vi "HeatFlow Conf Results.vi"(8 "error in":errorcluster, 9 "All signals?":bool, 11 "HW Cfg In":T2) -> (0 "error out":errorcluster, 2 "HeatFlowRes Cfg":T1, 3 "HW Cfg Out":T2)   [LabVIEW 2019, in "Acquisition.lvlib"]
uses:
  Acquisition.lvlib
  HeatFlow HW Cfg.ctl
  Logging/HeatFlow/HeatFlow Res Cfg.ctl
  Logging/HeatFlow/HeatFlow Results States.ctl
  Logging/Logging.lvlib
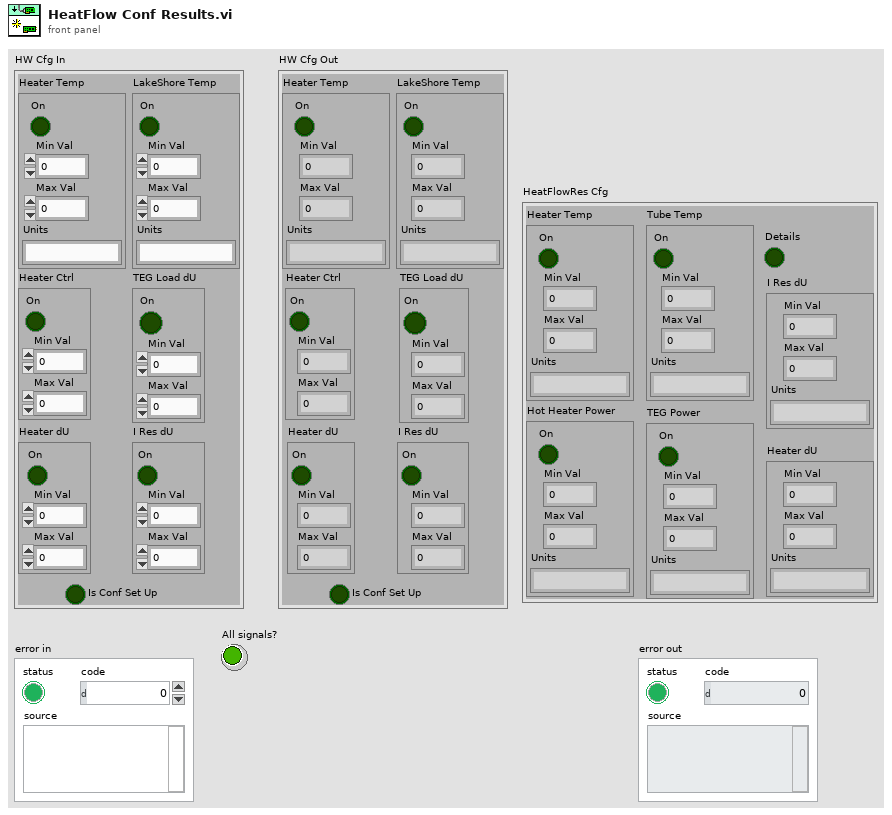
[diagram p1: front panel]
types:
  T1 = typedef "Logging.lvlib/HeatFlow Res Cfg.ctl" = cluster{"Heater Temp":cluster{"On":bool, "Min Val":dbl, "Max Val":dbl, "Units":string}, "Tube Temp":cluster{"On":bool, "Min Val":dbl, "Max Val":dbl, "Units":string}, "Hot Heater Power":cluster{"On":bool, "Min Val":dbl, "Max Val":dbl, "Units":string}, "TEG Power":cluster{"On":bool, "Min Val":dbl, "Max Val":dbl, "Units":string}, "Details":bool, "Heater dU":cluster{"Min Val":dbl, "Max Val":dbl, "Units":string}, "I Res dU":cluster{"Min Val":dbl, "Max Val":dbl, "Units":string}}
  T2 = typedef "Acquisition.lvlib/HeatFlow HW Cfg.ctl" = cluster{"Heater Temp":cluster{"On":bool, "Min Val":dbl, "Max Val":dbl, "Units":string}, "LakeShore Temp":cluster{"On":bool, "Min Val":dbl, "Max Val":dbl, "Units":string}, "Heater Ctrl":cluster{"On":bool, "Min Val":dbl, "Max Val":dbl}, "TEG Load dU":cluster{"On":bool, "Min Val":dbl, "Max Val":dbl}, "Heater dU":cluster{"On":bool, "Min Val":dbl, "Max Val":dbl}, "I Res dU":cluster{"On":bool, "Min Val":dbl, "Max Val":dbl}, "Is Conf Set Up":bool}
  T3 = typedef "Logging.lvlib/HeatFlow Results States.ctl" = enum16{"Start", "Timestamp", "Heater Temp", "Tube Temp", "Heater Power", "TEG Power", "Details", "End"}
  T4 = cluster{"On":bool, "Min Val":dbl, "Max Val":dbl, "Units":string}
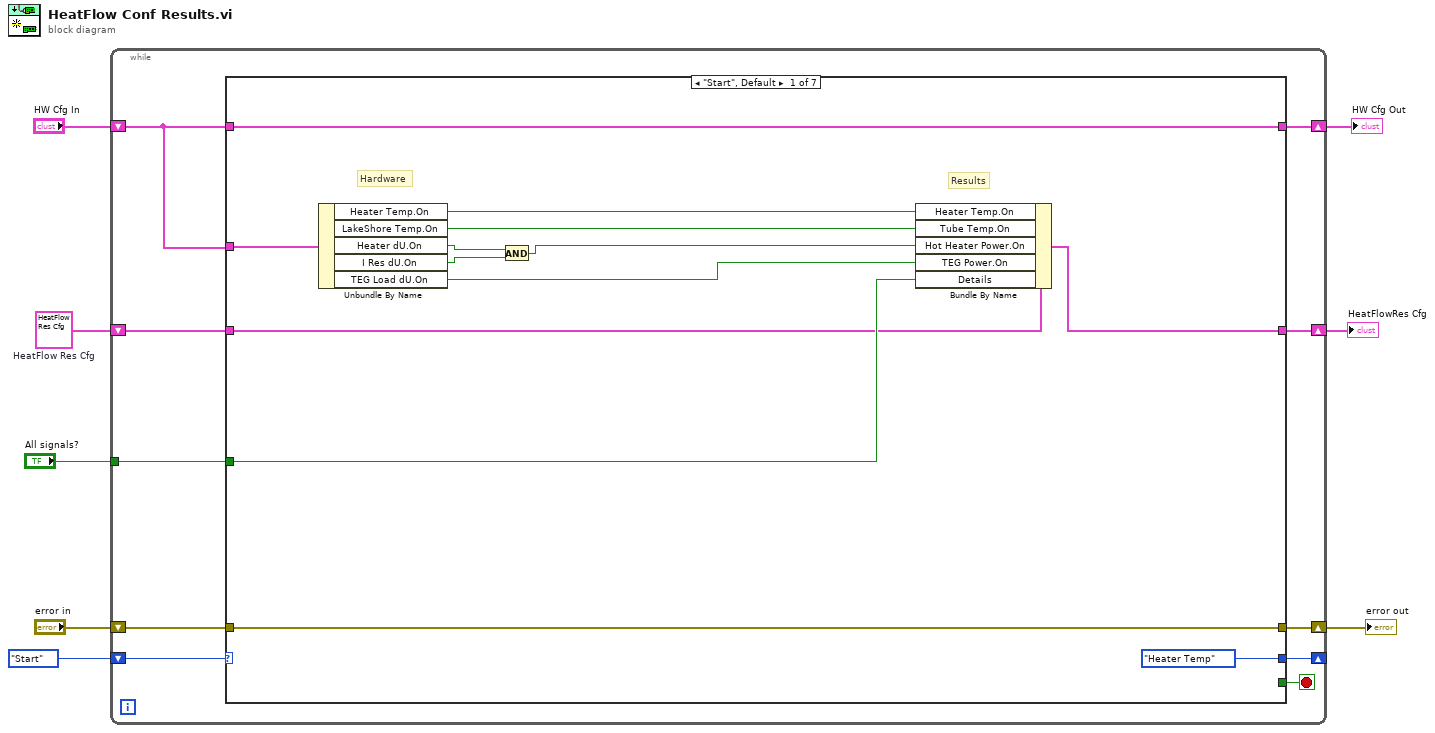
[diagram p0: block diagram]
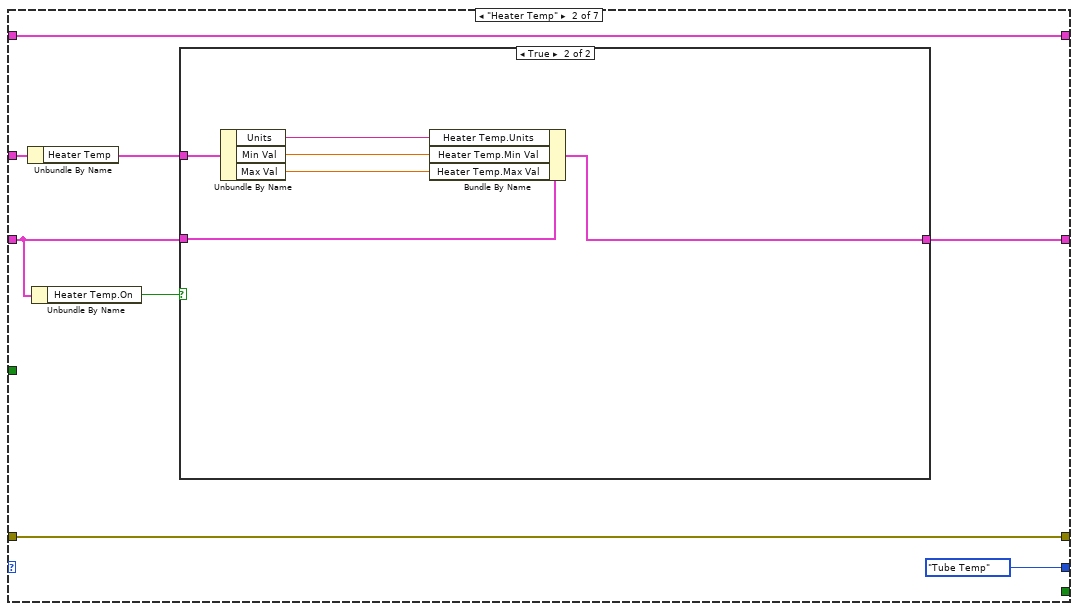
[diagram p2: hidden frame]
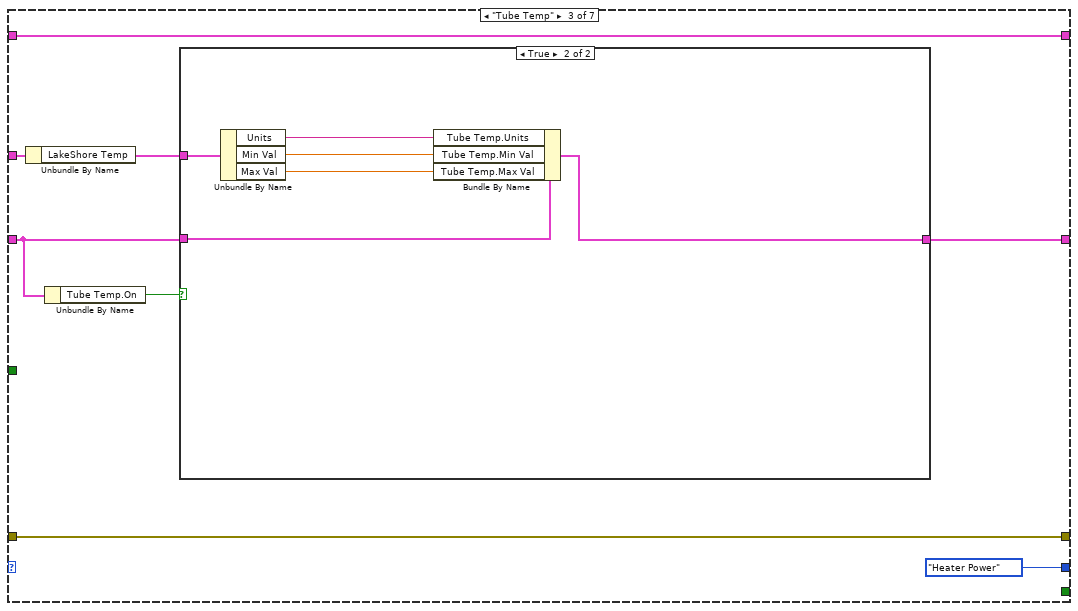
[diagram p4: hidden frame]
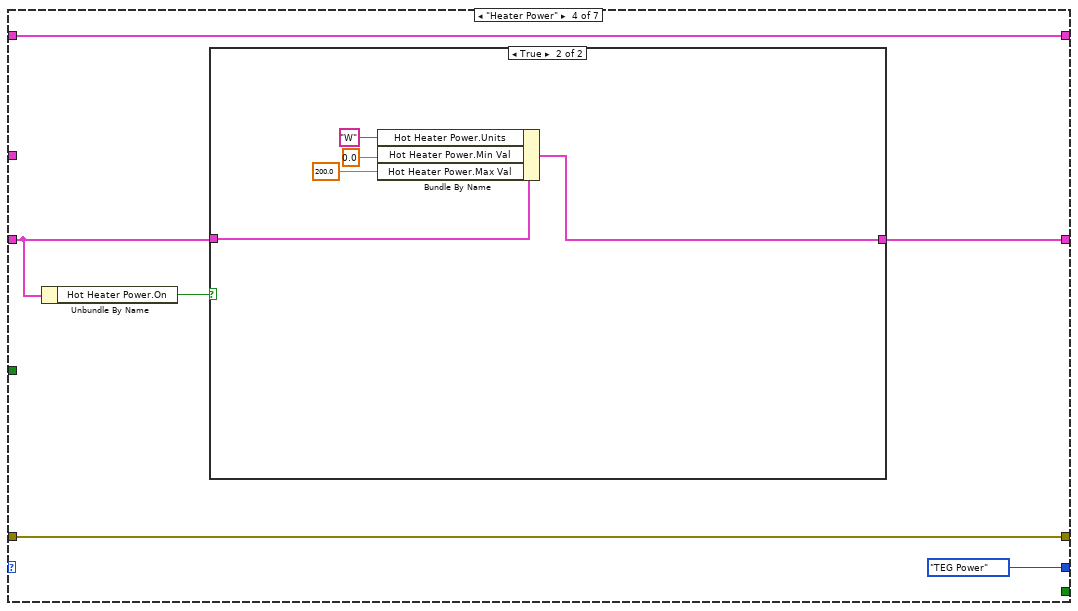
[diagram p6: hidden frame]
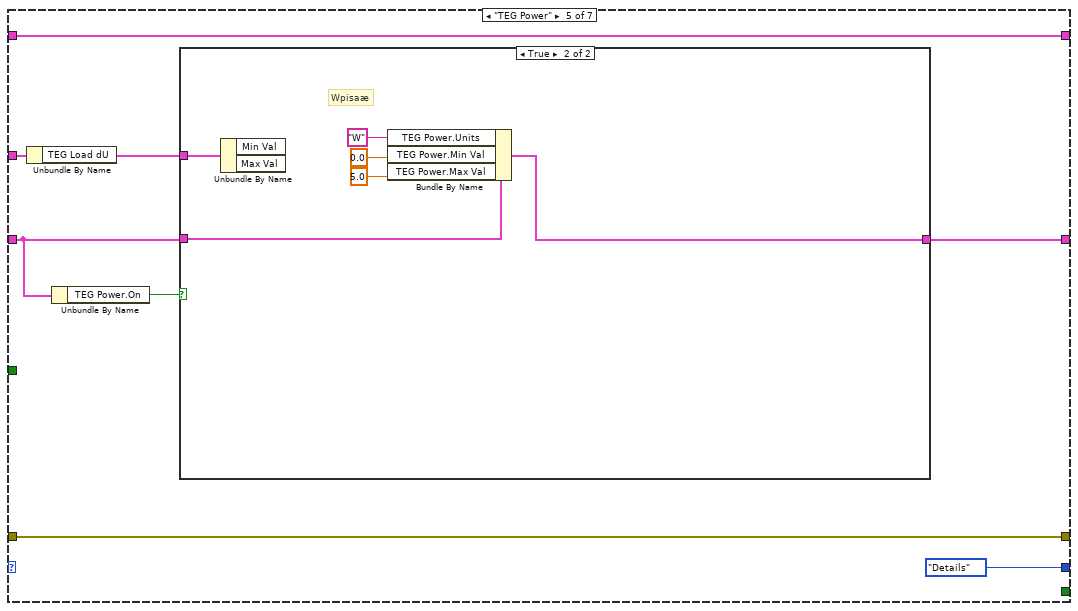
[diagram p8: hidden frame]
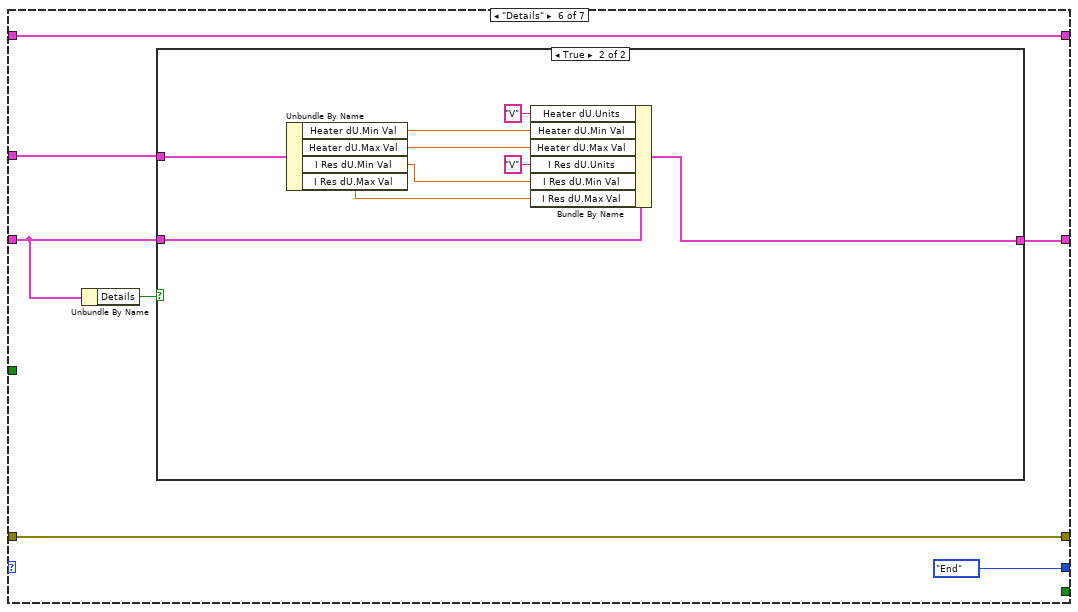
[diagram p10: hidden frame]
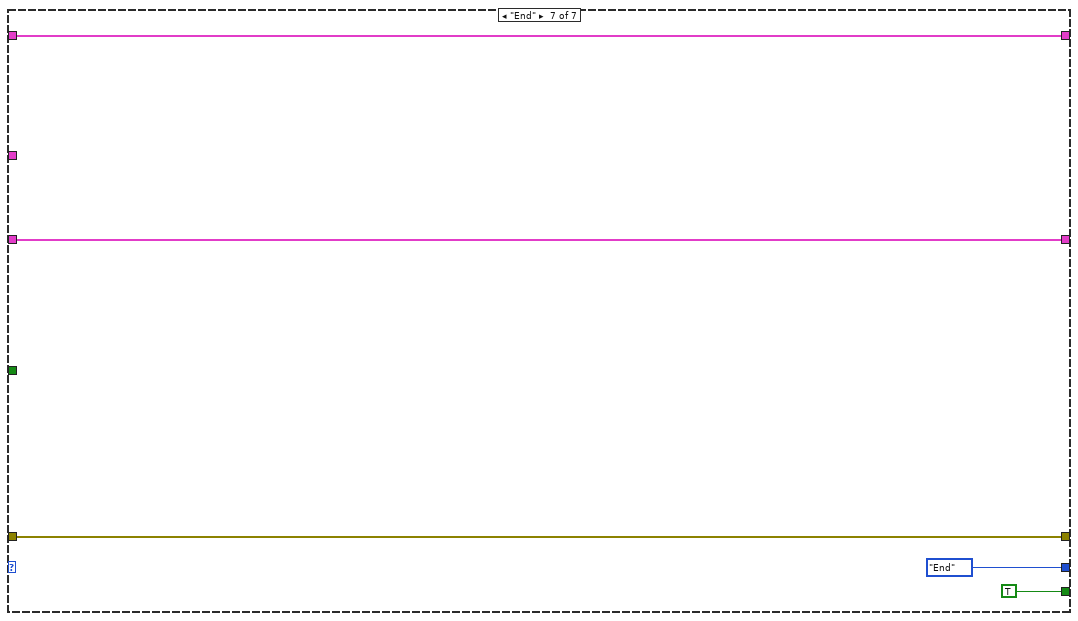
[diagram p12: hidden frame]
diagram:
  w2 = T1 {"Heater Temp"={"On"=FALSE, "Min Val"=0.0, "Max Val"=0.0, "Units"=""}, "Tube Temp"={"On"=FALSE, "Min Val"=0.0, "Max Val"=0.0, "Units"=""}, "Hot Heater Power"={"On"=FALSE, "Min Val"=0.0, "Max Val"=0.0, "Units"=""}, "TEG Power"={"On"=FALSE, "Min Val"=0.0, "Max Val"=0.0, "Units"=""}, "Details"=FALSE, "Heater dU"={"Min Val"=0.0, "Max Val"=0.0, "Units"=""}, "I Res dU"={"Min Val"=0.0, "Max Val"=0.0, "Units"=""}}  # HeatFlow Res Cfg
  n1 = while {
    shift-right: [w17] -> _
    shift-left: HeatFlow_Results_States."Start" ("Results") -> [w18]
    shift-right: [w16] -> w3
    shift-left: "HW Cfg In" -> [w11]
    shift-right: [w14] -> w5
    shift-left: "error in" -> [w15]
    tunnel: "All signals?" -> [w12]
    shift-right: [w9] -> w1
    shift-left: w2 -> [w10]
    stop <- w13 stop-if-true
    n2 = case shown="\"Start\", Default" w18 {
      tunnel: [HeatFlow_Results_States."Heater Temp" ("Results") HeatFlow_Results_States."Tube Temp" ("Results") HeatFlow_Results_States."Heater Power" ("Results") HeatFlow_Results_States."TEG Power" ("Results") HeatFlow_Results_States."Details" ("Results") HeatFlow_Results_States."End" ("Results") HeatFlow_Results_States."End" ("Results")] -> w17
      tunnel: w11 -> [w21 w33 w48 w63 w75 w93 w110]
      tunnel: [w21 w33 w48 w63 w75 w93 w110] -> w16
      tunnel: w15 -> [w31 w32 w47 w62 w74 w94 w109]
      tunnel: [w31 w32 w47 w62 w74 w94 w109] -> w14
      tunnel: w10 -> [w20 w36 w51 w65 w78 w91 w106]
      tunnel: [_ _ _ _ _ _ TRUE] -> w13
      tunnel: w12 -> [w28 _ _ _ _ _ _]
      tunnel: w11 -> [w27 w39 w54 _ w81 w92 _]
      tunnel: [w19 w34 w49 w64 w76 w89 w106] -> w9
      frame "Start", Default {
        # "Results"
        # "Hardware"
        n3 = Unbundle By Name(w27) -> ("Heater Temp.On"=w30:bool, "LakeShore Temp.On"=w29:bool, "Heater dU.On"=w25:bool, "I Res dU.On"=w24:bool, "TEG Load dU.On"=w22:bool)
        n4 = And(x=w25, y=w24) -> (x .and. y?=w23:bool)
        n5 = Bundle By Name(cluster=w20, "Heater Temp.On"=w30, "Tube Temp.On"=w29, "Hot Heater Power.On"=w23, "TEG Power.On"=w22, "Details"=w28) -> (w19:T1)
      }
      frame "Heater Temp" {
        n6 = Unbundle By Name(w39) -> ("Heater Temp"=w38:T4)
        n7 = Unbundle By Name(w36) -> ("Heater Temp.On"=w37:bool)
        n8 = case shown="True" w37 {
          tunnel: w38 -> [_ w46]
          tunnel: w36 -> [w40 w42]
          tunnel: [w40 w41] -> w34
          frame False {
            # "Inlet temperature measurement is off."
          }
          frame True {
            # "Inlet temperature measurement is on."
            n9 = Unbundle By Name(w46) -> ("Units"=w45:string, "Min Val"=w44:dbl, "Max Val"=w43:dbl)
            n10 = Bundle By Name(cluster=w42, "Heater Temp.Units"=w45, "Heater Temp.Min Val"=w44, "Heater Temp.Max Val"=w43) -> (w41:T1)
          }
        }
      }
      frame "Tube Temp" {
        n11 = Unbundle By Name(w54) -> ("LakeShore Temp"=w53:T4)
        n12 = Unbundle By Name(w51) -> ("Tube Temp.On"=w52:bool)
        n13 = case shown="True" w52 {
          tunnel: w53 -> [_ w61]
          tunnel: w51 -> [w55 w60]
          tunnel: [w55 w56] -> w49
          frame False {
            # "Inlet temperature measurement is off."
          }
          frame True {
            # "Inlet temperature measurement is on."
            n14 = Unbundle By Name(w61) -> ("Units"=w59:string, "Min Val"=w58:dbl, "Max Val"=w57:dbl)
            n15 = Bundle By Name(cluster=w60, "Tube Temp.Units"=w59, "Tube Temp.Min Val"=w58, "Tube Temp.Max Val"=w57) -> (w56:T1)
          }
        }
      }
      frame "Heater Power" {
        n16 = Unbundle By Name(w65) -> ("Hot Heater Power.On"=w67:bool)
        n17 = case shown="True" w67 {
          tunnel: w65 -> [w68 w73]
          tunnel: [w68 w69] -> w64
          frame False {
            # "Inlet temperature measurement is off."
          }
          frame True {
            # "Inlet temperature measurement is on."
            n18 = Bundle By Name(cluster=w73, "Hot Heater Power.Units"="W" ("Units"), "Hot Heater Power.Min Val"=0.0 ("Min Val"), "Hot Heater Power.Max Val"=200.0 ("Max Val")) -> (w69:T1)
          }
        }
      }
      frame "TEG Power" {
        n19 = Unbundle By Name(w81) -> ("TEG Load dU"=w80:cluster{"On":bool, "Min Val":dbl, "Max Val":dbl})
        n20 = Unbundle By Name(w78) -> ("TEG Power.On"=w79:bool)
        n21 = case shown="True" w79 {
          tunnel: w80 -> [_ w88]
          tunnel: w78 -> [w82 w87]
          tunnel: [w82 w83] -> w76
          frame False {
            # "Inlet temperature measurement is off."
          }
          frame True {
            # "Wpisaæ"
            # "Inlet temperature measurement is on."
            n22 = Unbundle By Name(w88) -> ()  [unwired: 2 out]
            n23 = Bundle By Name(cluster=w87, "TEG Power.Units"="W" ("Units"), "TEG Power.Min Val"=0.0 ("Min Val"), "TEG Power.Max Val"=5.0 ("Max Val")) -> (w83:T1)
          }
        }
      }
      frame "Details" {
        n24 = Unbundle By Name(w91) -> ("Details"=w90:bool)
        n25 = case shown="True" w90 {
          tunnel: w92 -> [_ w105]
          tunnel: w91 -> [w96 w104]
          tunnel: [w96 w103] -> w89
          frame False {
            # "Inlet temperature measurement is off."
          }
          frame True {
            # "Inlet temperature measurement is on."
            n26 = Unbundle By Name(w105) -> ("Heater dU.Min Val"=w102:dbl, "Heater dU.Max Val"=w101:dbl, "I Res dU.Min Val"=w100:dbl, "I Res dU.Max Val"=w99:dbl)
            n27 = Bundle By Name(cluster=w104, "Heater dU.Units"="V", "Heater dU.Min Val"=w102, "Heater dU.Max Val"=w101, "I Res dU.Units"="V", "I Res dU.Min Val"=w100, "I Res dU.Max Val"=w99) -> (w103:T1)
          }
        }
      }
      frame "End" {
      }
    }
  }
  "error out" <- w5
  "HW Cfg Out" <- w3
  "HeatFlowRes Cfg" <- w1
